vi "UI Loop Main.vi"(10 "UI Panel Ref":T1, 11 "Main Process Class out":refnum<class "Main Class.lvclass">) -> ()   [LabVIEW 2019]
uses:
  Class/Main Process Class/Main Class.lvclass
  LLB/Commonly VI/Ctrl/IDLevel.ctl
  LLB/Commonly VI/Main Glb.vi
  LLB/Message/main/MsgLog.vi
  IO Folder/IO_VI/IOCtrl/Ctrl/IO Card_Type.ctl
  LLB/Message/MsgShowAndLog.lvlib
  LLB/Commonly VI.lvlib
  Axis/Axis_Class/AxisCard.lvclass
  IO Folder/IO_Class/IOCard.lvclass
panel:
  in  "Tab Main 3":refnum<vi>
  in  "Tab Main":refnum<vi>
  out "error out 2":errorcluster
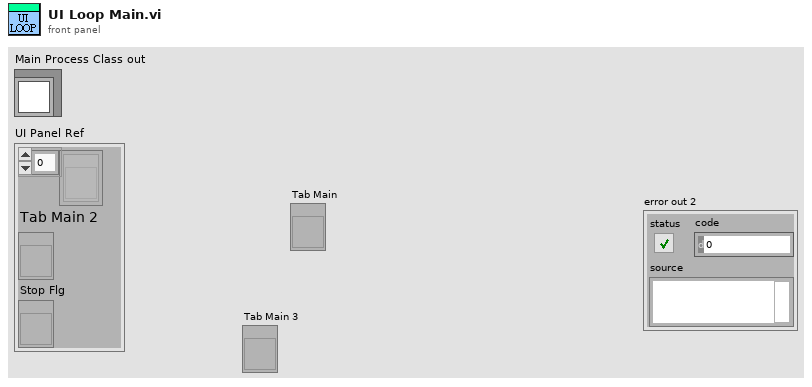
[diagram p1: front panel]
types:
  T1 = cluster{refnum<vi>[], "Tab Main 2":refnum<vi>, "Stop Flg":refnum<vi>}
  T2 = enum16{"initial", "Add", "Write", "Replace", "Delete", "REad"}
  T3 = typedef "IDLevel.ctl" = enum16{"Administrator", "Engineer", "Operator", "LogIn/Out"}
  T4 = typedef "IO Card_Type.ctl" = enum16{"None", "Unidaq32", "6480", "2410C-64", "Zan", "DMC1000B", "16InOut", "Robot", "DMC3600"}
  T5 = enum8{"Enabled", "Disabled", "Disabled and Grayed Out"}
  T6 = typedef "LVPointTypeDef.ctl" = cluster{"Horizontal":i16, "Vertical":i16}
  T7 = cluster{"AutoRunFlg":refnum<vi>, "Action Finish Flg":refnum<vi>, "Remaining Action":refnum<vi>, "Btn_AutoRun":refnum<vi>, "Manual Flg":refnum<vi>, "Sub Process Error":refnum<vi>}
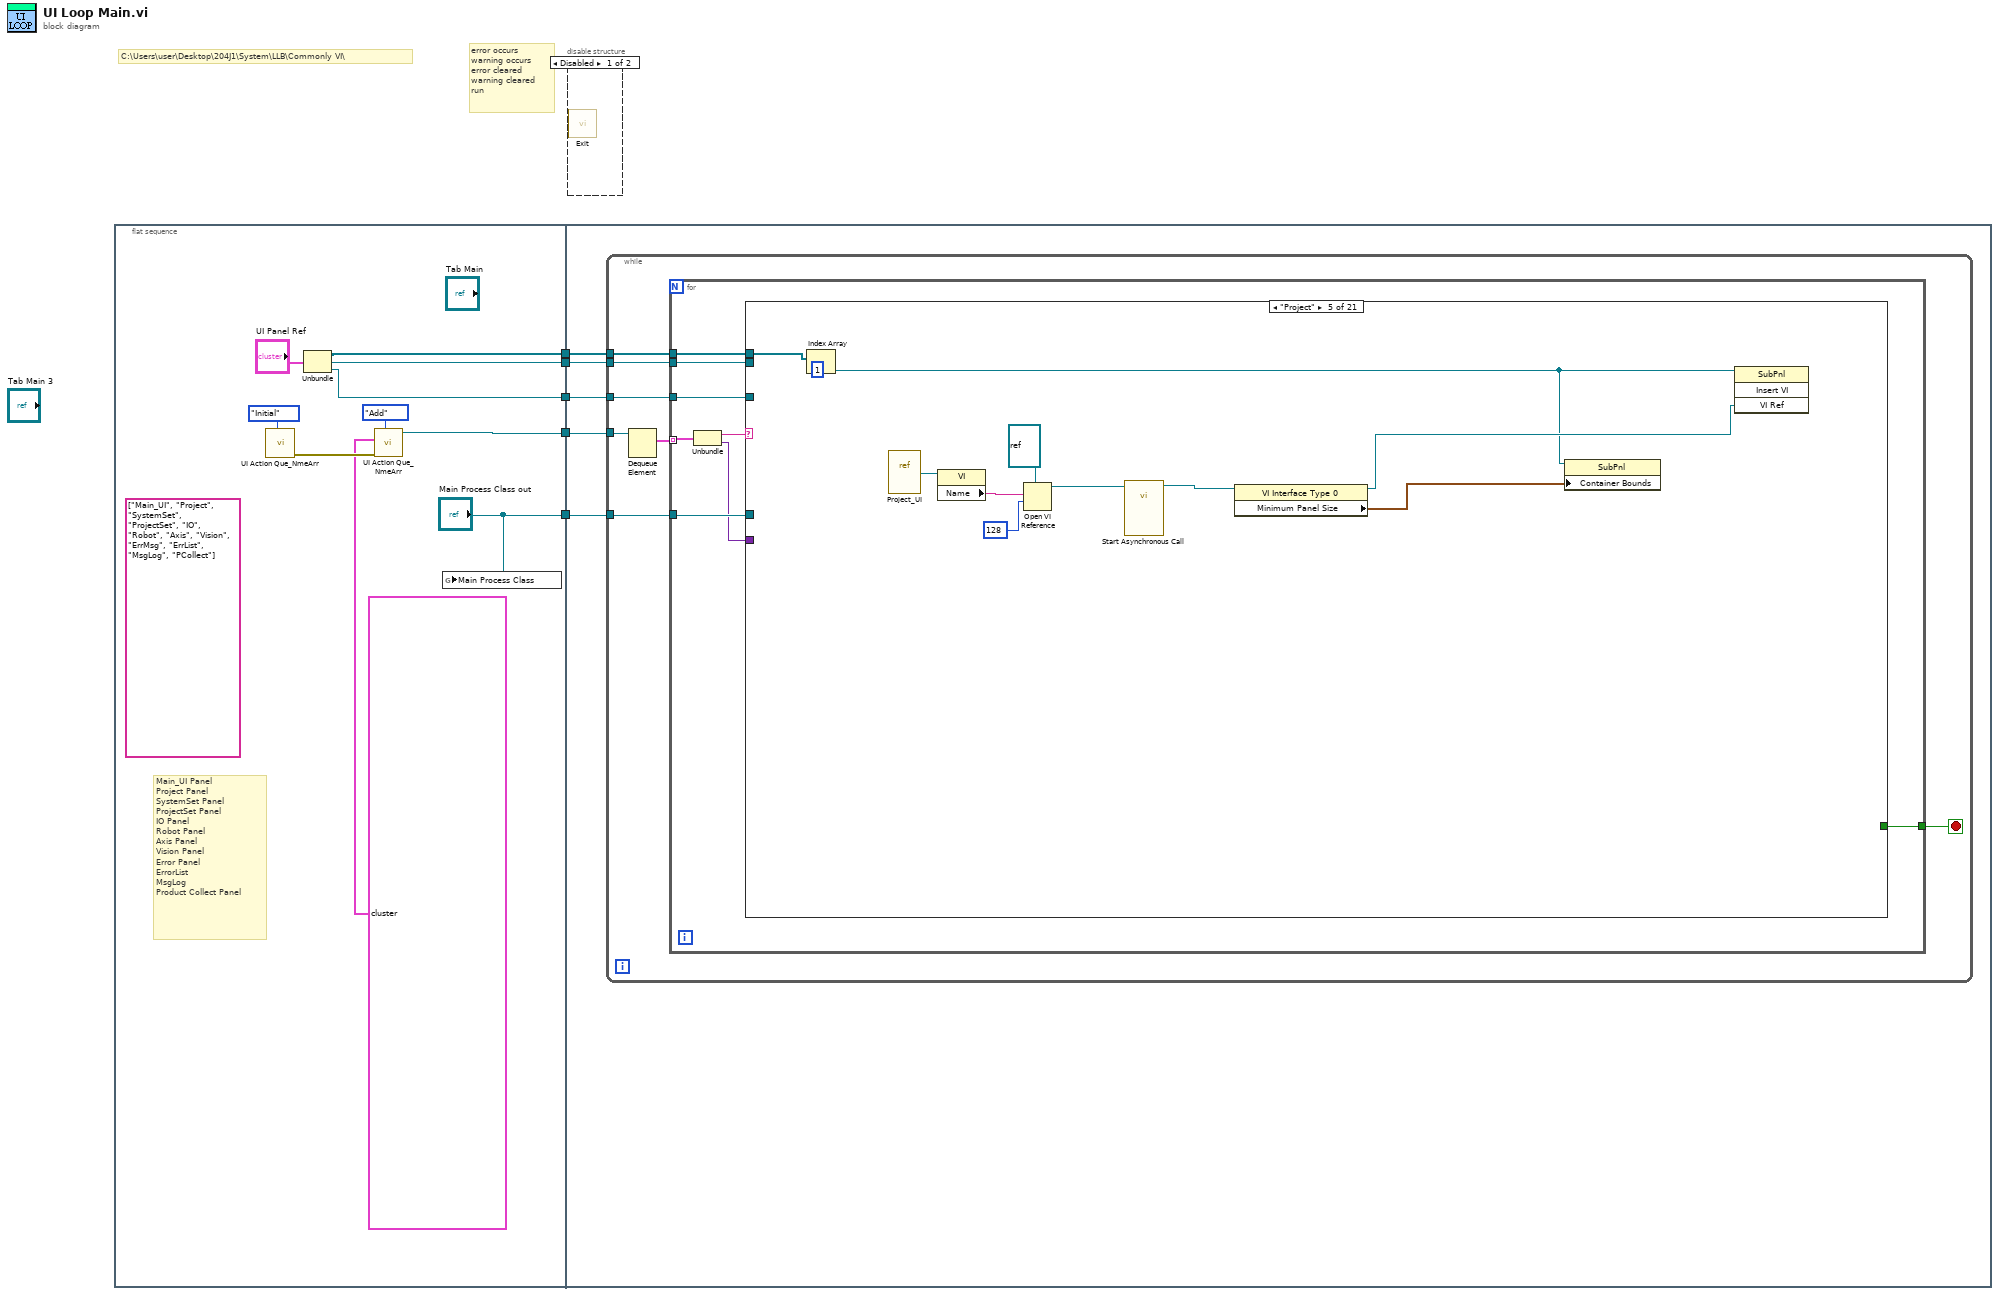
[diagram p0: block diagram]
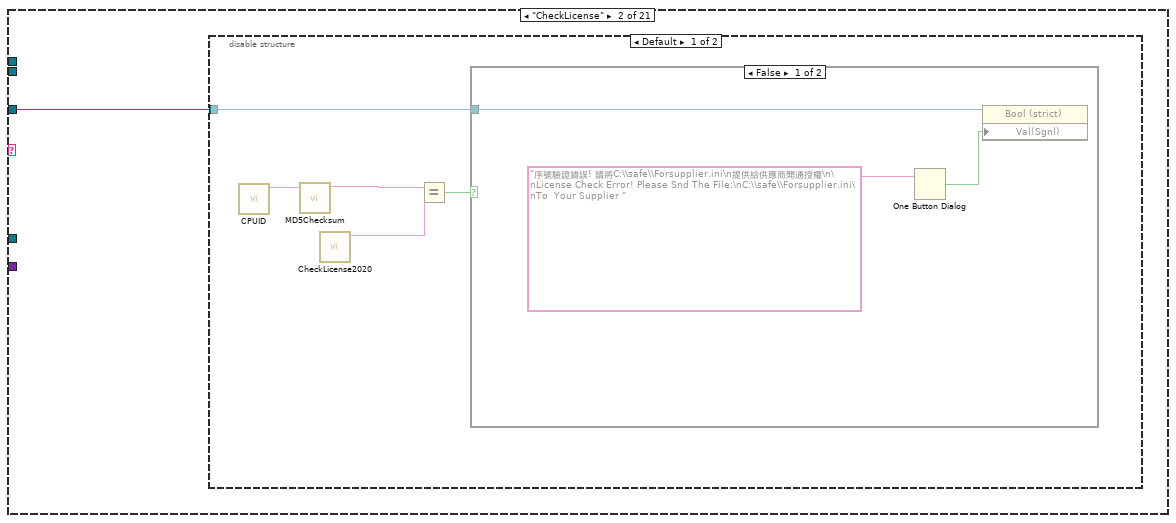
[diagram p4: hidden frame]
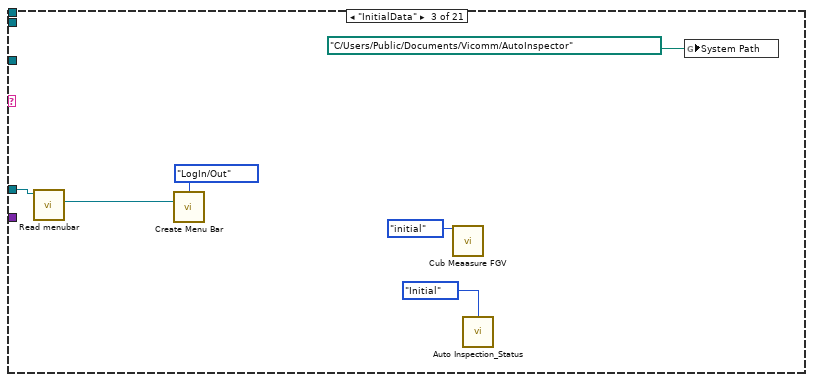
[diagram p7: hidden frame]
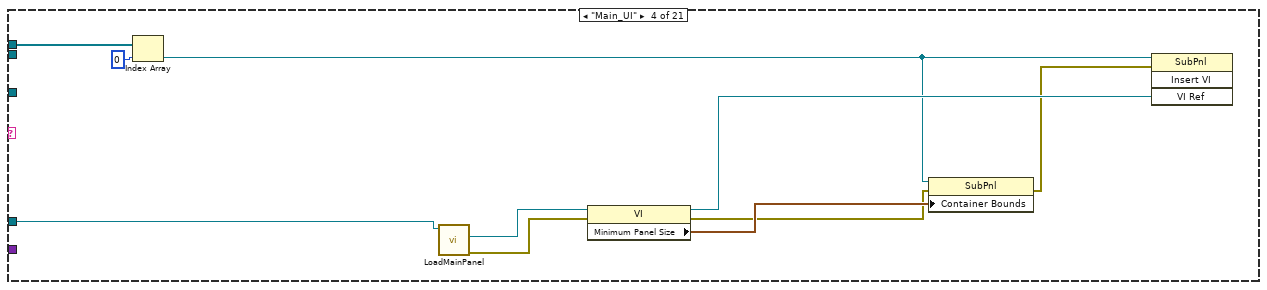
[diagram p8: hidden frame]
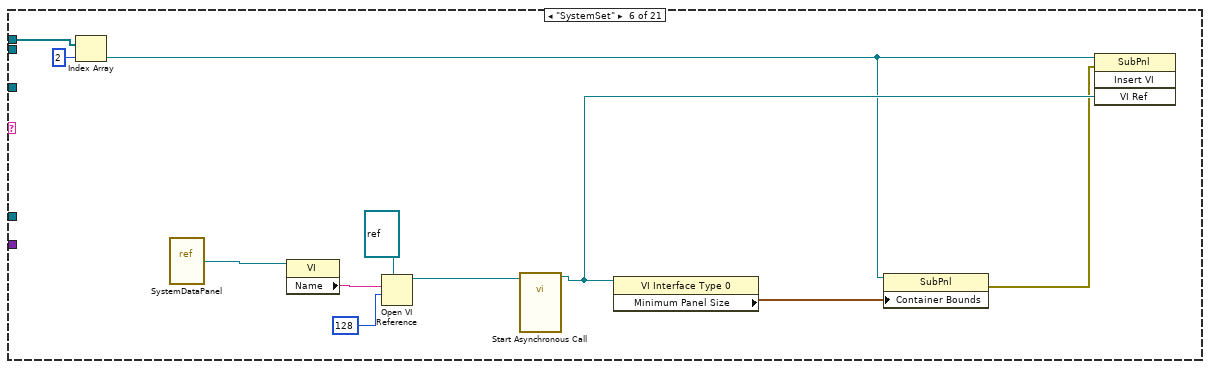
[diagram p9: hidden frame]
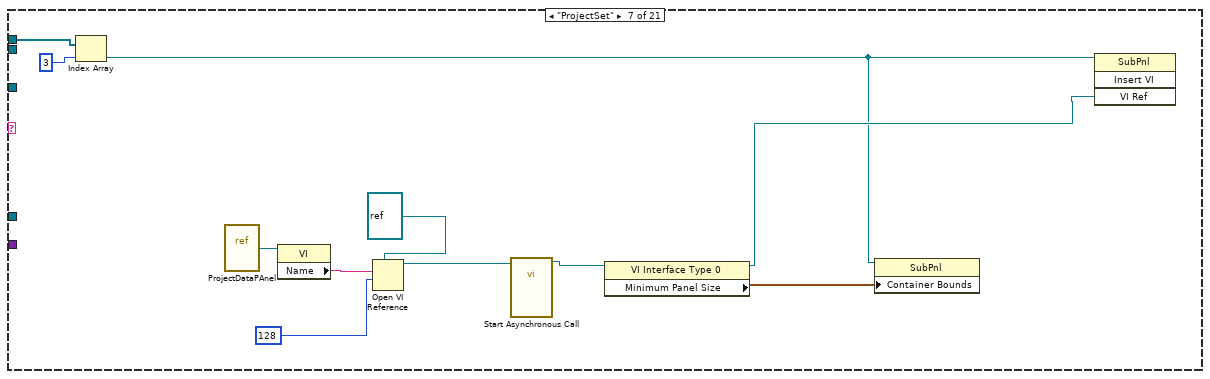
[diagram p10: hidden frame]
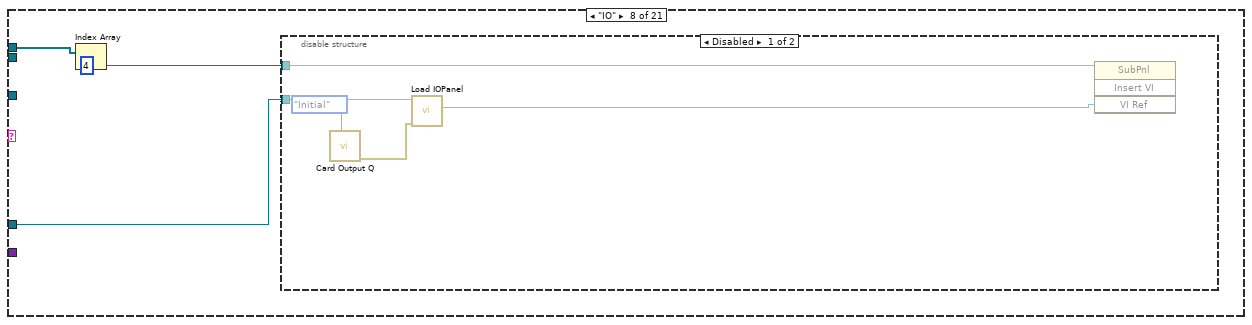
[diagram p11: hidden frame]
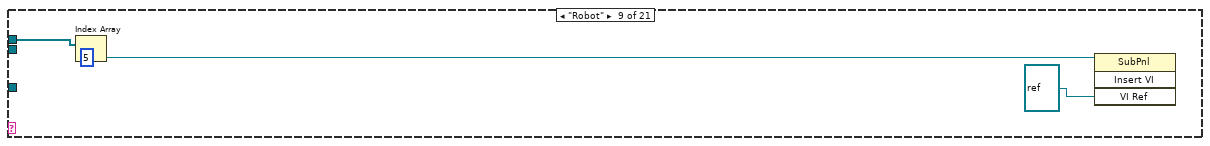
[diagram p13: hidden frame]
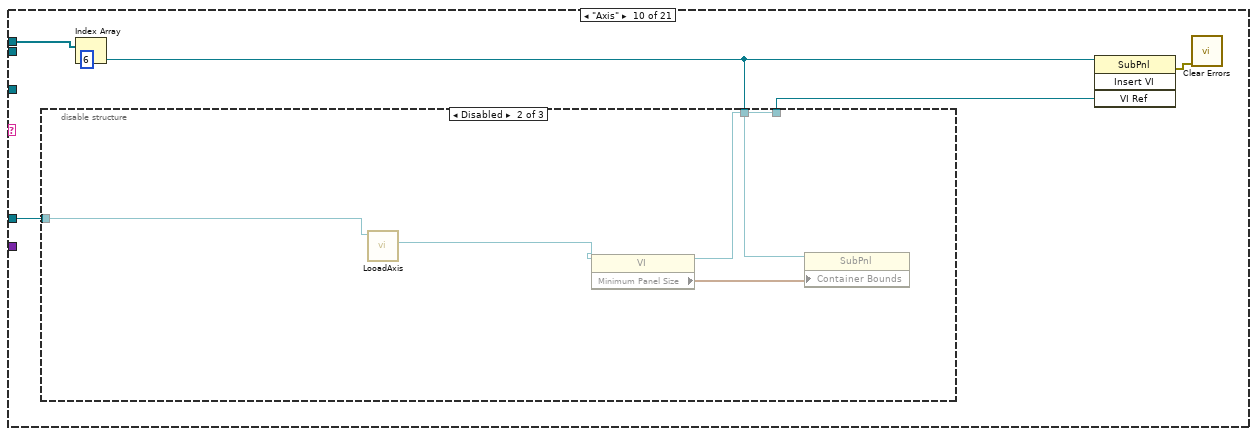
[diagram p14: hidden frame]
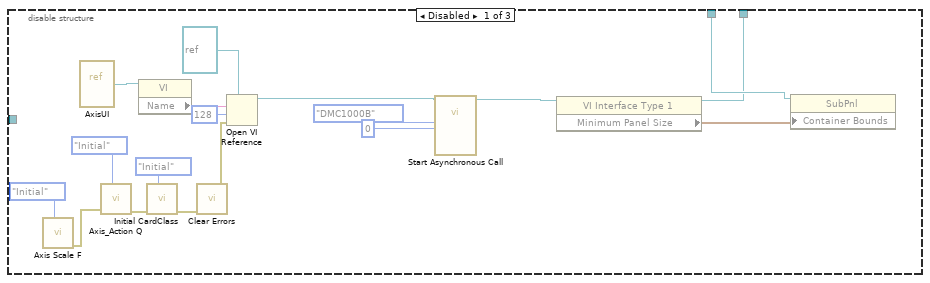
[diagram p15: hidden frame]
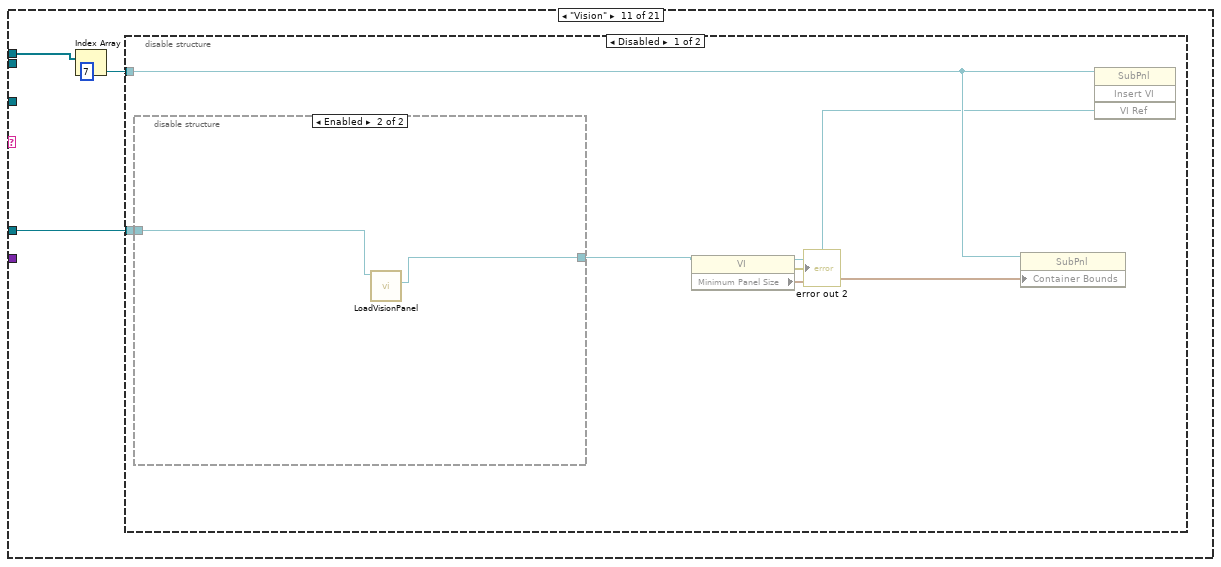
[diagram p17: hidden frame]
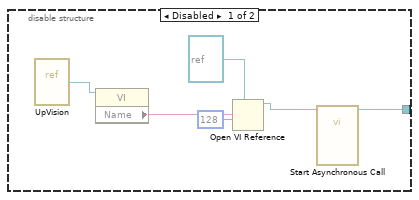
[diagram p18: hidden frame]
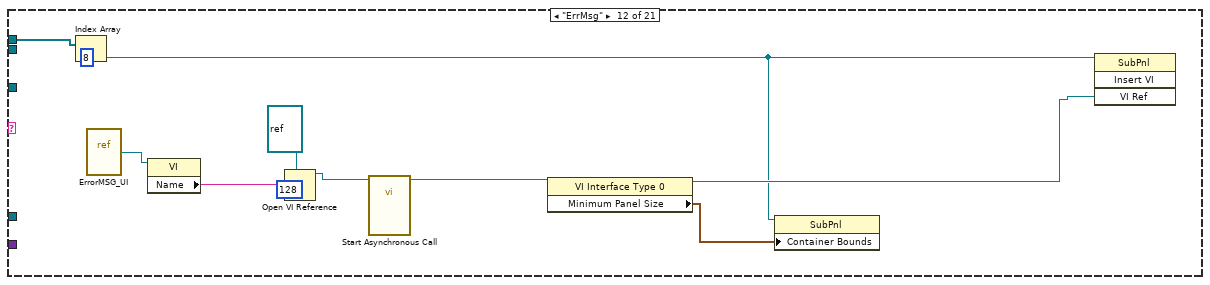
[diagram p20: hidden frame]
diagram:
  # "C:\\Users\\user\\Desktop\\204J1\\System\\LLB\\Commonly VI\\"
  # "error occurs\nwarning occurs\nerror cleared\nwarning cleared\nrun"
  n1 = flat-sequence {
    tunnel: [w13] -> w5
    tunnel: [w9] -> w4
    tunnel: [w8] -> w3
    tunnel: ["Main Process Class out"] -> w2
    tunnel: [w7] -> w1
    tunnel: w5 -> [w20]
    tunnel: w4 -> [w19]
    tunnel: w3 -> [w18]
    tunnel: w2 -> [w17]
    tunnel: w1 -> [w16]
    frame #0 {
      (unwired) string[] ["Main_UI", "Project", "SystemSet", "ProjectSet", "IO", "Robot", "Axis", "Vision", "ErrMsg", "ErrList", "MsgLog", "PCollect"] ("UI Process")
      # "Main_UI Panel\nProject Panel\nSystemSet Panel\nProjectSet Panel\nIO Panel\nRobot Panel\nAxis Panel\nVision Panel\nError Panel\nErrorList\nMsgLog\nProduct Collect Panel"
      n2 = call "UI Action Que_NmeArr.vi"("Action"=enum16{"Initial", "Add", "Release"}."Initial") -> ("error out"=w12:errorcluster)  [unwired: 9 in, 1 out]
      n3 = Unbundle("UI Panel Ref") -> (w9:refnum<vi>[], "Tab Main 2"=w8:refnum<vi>, "Stop Flg"=w7:refnum<vi>)
      n4 = call "UI Action Que_NmeArr.vi"("Action"=enum16{"Initial", "Add", "Release"}."Add", "error in (no error)"=w12, "UI Process"=cluster{"Action":string, "Value":variant}[] [{"Action"="CheckLicense", "Value"=variant}, {"Action"="InitialData", "Value"=variant}, {"Action"="Main_UI", "Value"=variant}, {"Action"="ErrMsg", "Value"=variant}, {"Action"="MsgLog", "Value"=variant}, {"Action"="Project", "Value"=variant}, {"Action"="SystemSet", "Value"=variant}, {"Action"="ProjectSet", "Value"=variant}, {"Action"="IO", "Value"=variant}, {"Action"="Axis", "Value"=variant}, {"Action"="Vision", "Value"=variant}, {"Action"="ErrList", "Value"=variant}, {"Action"="MsgLog", "Value"=variant}, {"Action"="PCollect", "Value"=variant}, {"Action"="Prevention Panel", "Value"=variant}]) -> ("Process Que Out"=w13:refnum<queue>)  [unwired: 7 in, 1 out]
      n5 = global write "Main Glb.vi" "Main Process Class"("Main Process Class out") -> ()
    }
    frame #1 {
      n6 = while {
        tunnel: w20 -> [w27]
        tunnel: w19 -> [w24]
        tunnel: w18 -> [w22]
        tunnel: w17 -> [w23]
        tunnel: w16 -> [w21]
        stop <- w25 stop-if-true
        n7 = Dequeue Element(queue=w27) -> (element=w26:cluster{"Action":string, "Value":variant}[])  [unwired: 2 in, 3 out]
        n8 = for {
          tunnel: w26 -> [w33] mode=indexing
          tunnel: [w35] -> w25
          tunnel: w24 -> [w34]
          tunnel: w23 -> [w31]
          tunnel: w22 -> [w29]
          tunnel: w21 -> [w28]
          n9 = Unbundle(w33) -> ("Action"=w32:string, "Value"=w30:variant)
          n10 = case shown="\"Project\"" w32 {
            tunnel: [_ _ _ _ _ _ _ _ _ _ _ _ _ _ _ _ _ _ _ _ TRUE] -> w35
            tunnel: w34 -> [_ _ _ w60 w70 w81 w92 w95 w104 w111 w138 w163 w171 w183 w195 w204 _ _ _ _ _]
            tunnel: w31 -> [_ _ w49 w55 _ _ _ w94 _ w108 w136 _ w165 _ _ _ w221 _ w230 w236 _]
            tunnel: w30 -> [_ _ _ _ _ _ _ _ _ _ _ _ _ _ _ _ w219 w224 w227 w233 _]
            tunnel: w29 -> [_ _ _ _ _ _ _ _ _ _ _ _ _ _ _ _ w216 w225 _ _ _]
            tunnel: w28 -> [_ w36 _ _ _ _ _ _ _ _ _ _ _ _ _ _ _ _ _ _ _]
            frame Default {
            }
            frame "CheckLicense" {
              n11 = disable-structure shown="Default" {
                disable-tunnel: w36 -> [w41 _]
                frame condition #0 {
                  n12 = call "CPUID.vi"() -> ("ToString"=w40:string)  [unwired: 11 in]
                  n13 = call "MD5Checksum.vi"("Message String"=w40) -> ("MD5 message-digest"=w37:string)  [unwired: 10 in]
                  n14 = call "CheckLicense2020.vi"() -> ("CPU"=w38:string)  [unwired: 11 in]
                  n15 = Equal?(x=w37, y=w38) -> (x = y?=w39:bool)
                  n16 = case shown="False" w39 {
                    tunnel: w41 -> [w44 _]
                    frame False {
                      n17 = One Button Dialog(message="序號驗證錯誤! 請將C:\\safe\\Forsupplier.ini\n提供給供應商開通授權\n\nLicense Check Error! Please Snd The File:\nC:\\safe\\Forsupplier.ini\nTo  Your Supplier ") -> (true=w42:bool)  [unwired: 1 in]
                      n18 = property class="Bool (strict)"(reference=w44, "Val(Sgnl)"=w42) -> ()  [unwired: 1 in, 2 out]
                    }
                    frame True {
                    }
                  }
                }
                frame condition #1 (active) {
                }
              }
            }
            frame "InitialData" {
              n19 = call-dynamic "Read menubar.vi"("Main Class in"=w49) -> ("menubar"=w48:refnum<k9>)  [unwired: 8 in, 2 out]
              n20 = call "Create Menu Bar.vi"("Entry Level"=IDLevel."LogIn/Out", "menubar"=w48) -> ()  [unwired: 13 in, 1 out]
              n21 = call "Cub Meaasure FGV.vi"("Action"=T2."initial" ("Enum")) -> ()  [unwired: 11 in, 8 out]
              n22 = call "Auto Inspection_Status.vi"("Action"=enum16{"Initial", "Write", "Read"}."Initial") -> ()  [unwired: 12 in, 3 out]
              n23 = global write "Main Glb.vi" "System Path"(path "C:/Users/Public/Documents/Vicomm/AutoInspector" ("path")) -> ()
            }
            frame "Main_UI" {
              n24 = Index Array(array=w60, index=0) -> (element=w56:refnum<vi>)
              n25 = call-dynamic "LoadMainPanel.vi"("Main Class in"=w55) -> ("error out"=w54:errorcluster, "This VI"=w51:refnum<vi>)  [unwired: 8 in, 1 out]
              n26 = property class="VI"(reference=w51, error in=w54) -> (reference out=w57:refnum<vi>, error out=w53:errorcluster, "Minimum Panel Size"=w58:T6)
              n27 = property class="SubPnl"(reference=w56, error in=w53, "Container Bounds"=w58) -> (error out=w52:errorcluster)  [unwired: 1 out]
              n28 = invoke class="SubPnl" method="Insert VI"(reference=w56, error in=w52, "VI Ref"=w57) -> ()  [unwired: 1 in, 4 out]
            }
            frame "Project" {
              n29 = Index Array(array=w70, index=1) -> (element=w62:refnum<vi>)
              n30 = vi-ref "Project_UI.vi"() -> (w69:refnum<vi>)
              n31 = property class="VI"(reference=w69) -> ("Name"=w68:string)  [unwired: 1 in, 2 out]
              n32 = Open VI Reference(type specifier VI Refnum (for type only)=refnum<vi> refnum, vi path=w68, options=128) -> (vi reference=w67:refnum<vi>)  [unwired: 3 in, 1 out]
              n33 = call-by-ref "Start Asynchronous Call"(reference=w67) -> (reference out=w66:refnum<vi>)  [unwired: 13 in, 1 out]
              n34 = property class="VI Interface Type 0"(reference=w66) -> (reference out=w63:refnum<vi>, "Minimum Panel Size"=w65:T6)  [unwired: 1 in, 1 out]
              n35 = property class="SubPnl"(reference=w62, "Container Bounds"=w65) -> ()  [unwired: 1 in, 2 out]
              n36 = invoke class="SubPnl" method="Insert VI"(reference=w62, "VI Ref"=w63) -> ()  [unwired: 2 in, 4 out]
            }
            frame "SystemSet" {
              n37 = Index Array(array=w81, index=2) -> (element=w73:refnum<vi>)
              n38 = vi-ref "SystemDataPanel.vi"() -> (w80:refnum<vi>)
              n39 = property class="VI"(reference=w80) -> ("Name"=w79:string)  [unwired: 1 in, 2 out]
              n40 = Open VI Reference(type specifier VI Refnum (for type only)=refnum<vi> refnum, vi path=w79, options=128) -> (vi reference=w78:refnum<vi>)  [unwired: 3 in, 1 out]
              n41 = call-by-ref "Start Asynchronous Call"(reference=w78) -> (reference out=w74:refnum<vi>)  [unwired: 13 in, 1 out]
              n42 = property class="VI Interface Type 0"(reference=w74) -> ("Minimum Panel Size"=w77:T6)  [unwired: 1 in, 2 out]
              n43 = property class="SubPnl"(reference=w73, "Container Bounds"=w77) -> (error out=w72:errorcluster)  [unwired: 1 in, 1 out]
              n44 = invoke class="SubPnl" method="Insert VI"(reference=w73, error in=w72, "VI Ref"=w74) -> ()  [unwired: 1 in, 4 out]
            }
            frame "ProjectSet" {
              n45 = Index Array(array=w92, index=3) -> (element=w84:refnum<vi>)
              n46 = vi-ref "ProjectDataPAnel.vi"() -> (w83:refnum<vi>)
              n47 = property class="VI"(reference=w83) -> ("Name"=w91:string)  [unwired: 1 in, 2 out]
              n48 = Open VI Reference(type specifier VI Refnum (for type only)=refnum<vi> refnum, vi path=w91, options=128) -> (vi reference=w90:refnum<vi>)  [unwired: 3 in, 1 out]
              n49 = call-by-ref "Start Asynchronous Call"(reference=w90) -> (reference out=w88:refnum<vi>)  [unwired: 13 in, 1 out]
              n50 = property class="VI Interface Type 0"(reference=w88) -> (reference out=w85:refnum<vi>, "Minimum Panel Size"=w89:T6)  [unwired: 1 in, 1 out]
              n51 = property class="SubPnl"(reference=w84, "Container Bounds"=w89) -> ()  [unwired: 1 in, 2 out]
              n52 = invoke class="SubPnl" method="Insert VI"(reference=w84, "VI Ref"=w85) -> ()  [unwired: 2 in, 4 out]
            }
            frame "IO" {
              n53 = Index Array(array=w95, index=4) -> (element=w97:refnum<vi>)
              n54 = disable-structure shown="Disabled" {
                disable-tunnel: w97 -> [w102 _]
                disable-tunnel: w94 -> [w101 _]
                frame Disabled {
                  n55 = call "Card Output Q.vi"("Action"=enum16{"Initial", "Write", "Read", "Release"}."Initial") -> ("error Out"=w98:errorcluster)  [unwired: 9 in, 1 out]
                  n56 = call-dynamic "Load IOPanel.vi"("error in (no error)"=w98, "Main Class in"=w101) -> ("This VI"=w100:refnum<vi>)  [unwired: 7 in, 2 out]
                  n57 = invoke class="SubPnl" method="Insert VI"(reference=w102, "VI Ref"=w100) -> ()  [unwired: 2 in, 4 out]
                }
                frame Enabled {
                }
              }
            }
            frame "Robot" {
              n58 = Index Array(array=w104, index=5) -> (element=w106:refnum<vi>)
              n59 = invoke class="SubPnl" method="Insert VI"(reference=w106, "VI Ref"=refnum<vi> refnum) -> ()  [unwired: 2 in, 4 out]
            }
            frame "Axis" {
              n60 = Index Array(array=w111, index=6) -> (element=w110:refnum<vi>)
              n61 = disable-structure shown="Disabled" {
                disable-tunnel: w110 -> [w122 w133 _]
                disable-tunnel: [w120 w132 _] -> w109
                disable-tunnel: w108 -> [_ w135 _]
                frame Disabled {
                  n62 = call "Axis Scale F.vi"("Enum"=enum16{"Initial", "Read"}."Initial") -> ("error Out"=w115:errorcluster)  [unwired: 9 in, 1 out]
                  n63 = vi-ref "AxisUI.vi"() -> (w130:refnum<vi>)
                  n64 = call "Axis_Action Q.vi"("Enum"=enum16{"Initial", "Write", "Read"}."Initial", "error in"=w115) -> ("error out"=w117:errorcluster)  [unwired: 7 in, 2 out]
                  n65 = property class="VI"(reference=w130) -> ("Name"=w129:string)  [unwired: 1 in, 2 out]
                  n66 = call "Initial CardClass.vi"("Enum"=enum16{"Initial", "Write", "Read", "Exit"}."Initial", "error in"=w117) -> ("error Out"=w116:errorcluster)  [unwired: 8 in, 1 out]
                  n67 = call <vilib>:"Clear Errors.vi"("error in (no error)"=w116) -> ("error out"=w113:errorcluster)  [unwired: 5 in, 1 out]
                  n68 = Open VI Reference(type specifier VI Refnum (for type only)=refnum<vi> refnum, vi path=w129, options=128, error in (no error)=w113) -> (vi reference=w126:refnum<vi>)  [unwired: 2 in, 1 out]
                  n69 = call-by-ref "Start Asynchronous Call"(reference=w126, "CardNumber"=0, "IO Card Type"=IO_Card_Type."DMC1000B") -> (reference out=w123:refnum<vi>)  [unwired: 11 in, 1 out]
                  n70 = property class="VI Interface Type 1"(reference=w123) -> (reference out=w120:refnum<vi>, "Minimum Panel Size"=w121:T6)  [unwired: 1 in, 1 out]
                  n71 = property class="SubPnl"(reference=w122, "Container Bounds"=w121) -> ()  [unwired: 1 in, 2 out]
                }
                frame Disabled {
                  n72 = call-dynamic "LooadAxis.vi"("Main Class in"=w135) -> ("This VI"=w131:refnum<vi>)  [unwired: 8 in, 2 out]
                  n73 = property class="VI"(reference=w131) -> (reference out=w132:refnum<vi>, "Minimum Panel Size"=w134:T6)  [unwired: 1 in, 1 out]
                  n74 = property class="SubPnl"(reference=w133, "Container Bounds"=w134) -> ()  [unwired: 1 in, 2 out]
                }
                frame Enabled {
                }
              }
              n75 = invoke class="SubPnl" method="Insert VI"(reference=w110, "VI Ref"=w109) -> (error out=w107:errorcluster)  [unwired: 2 in, 3 out]
              n76 = call <vilib>:"Clear Errors.vi"("error in (no error)"=w107) -> ()  [unwired: 5 in, 2 out]
            }
            frame "Vision" {
              n77 = Index Array(array=w138, index=7) -> (element=w137:refnum<vi>)
              n78 = disable-structure shown="Disabled" {
                disable-tunnel: w137 -> [w143 _]
                disable-tunnel: w136 -> [w141 _]
                frame Disabled {
                  n79 = disable-structure shown="Enabled" {
                    disable-tunnel: [w148 w152] -> w145
                    disable-tunnel: w141 -> [_ w153]
                    frame Disabled {
                      n80 = vi-ref "UpVision.vi"() -> (w151:refnum<vi>)
                      n81 = property class="VI"(reference=w151) -> ("Name"=w150:string)  [unwired: 1 in, 2 out]
                      n82 = Open VI Reference(type specifier VI Refnum (for type only)=refnum<vi> refnum, vi path=w150, options=128) -> (vi reference=w149:refnum<vi>)  [unwired: 3 in, 1 out]
                      n83 = call-by-ref "Start Asynchronous Call"(reference=w149) -> (reference out=w148:refnum<vi>)  [unwired: 13 in, 1 out]
                    }
                    frame Enabled {
                      n84 = call-dynamic "LoadVisionPanel.vi"("Main Class in"=w153) -> ("This VI"=w152:refnum<vi>)  [unwired: 8 in, 2 out]
                    }
                  }
                  n85 = property class="VI"(reference=w145) -> (reference out=w142:refnum<vi>, error out=→"error out 2":errorcluster, "Minimum Panel Size"=w144:T6)  [unwired: 1 in]
                  n86 = property class="SubPnl"(reference=w143, "Container Bounds"=w144) -> ()  [unwired: 1 in, 2 out]
                  n87 = invoke class="SubPnl" method="Insert VI"(reference=w143, "VI Ref"=w142) -> ()  [unwired: 2 in, 4 out]
                }
                frame Enabled {
                }
              }
            }
            frame "ErrMsg" {
              n88 = Index Array(array=w163, index=8) -> (element=w155:refnum<vi>)
              n89 = vi-ref "ErrorMSG_UI.vi"() -> (w162:refnum<vi>)
              n90 = property class="VI"(reference=w162) -> ("Name"=w161:string)  [unwired: 1 in, 2 out]
              n91 = Open VI Reference(type specifier VI Refnum (for type only)=refnum<vi> refnum, vi path=w161, options=128) -> (vi reference=w158:refnum<vi>)  [unwired: 3 in, 1 out]
              n92 = call-by-ref "Start Asynchronous Call"(reference=w158) -> (reference out=w157:refnum<vi>)  [unwired: 13 in, 1 out]
              n93 = property class="VI Interface Type 0"(reference=w157) -> (reference out=w156:refnum<vi>, "Minimum Panel Size"=w154:T6)  [unwired: 1 in, 1 out]
              n94 = property class="SubPnl"(reference=w155, "Container Bounds"=w154) -> ()  [unwired: 1 in, 2 out]
              n95 = invoke class="SubPnl" method="Insert VI"(reference=w155, "VI Ref"=w156) -> ()  [unwired: 2 in, 4 out]
            }
            frame "ErrList" {
              n96 = Index Array(array=w171, index=9) -> (element=w169:refnum<vi>)
              n97 = call-dynamic "LoadAdvancePanel.vi"("Main Class in"=w165) -> ("This VI"=w167:refnum<vi>)  [unwired: 8 in, 2 out]
              n98 = property class="VI"(reference=w167) -> (reference out=w166:refnum<vi>, "Minimum Panel Size"=w170:T6)  [unwired: 1 in, 1 out]
              n99 = property class="SubPnl"(reference=w169, "Container Bounds"=w170) -> (reference out=w168:refnum<vi>)  [unwired: 1 in, 1 out]
              n100 = invoke class="SubPnl" method="Insert VI"(reference=w168, "VI Ref"=w166) -> ()  [unwired: 2 in, 4 out]
            }
            frame "MsgLog" {
              n101 = Index Array(array=w183, index=10) -> (element=w176:refnum<vi>)
              n102 = vi-ref "MsgShowAndLog.lvlib:MsgLog.vi"() -> (w182:refnum<vi>)
              n103 = property class="VI"(reference=w182) -> ("Name"=w181:string)  [unwired: 1 in, 2 out]
              n104 = Open VI Reference(type specifier VI Refnum (for type only)=refnum<vi> refnum, vi path=w181, options=128) -> (vi reference=w179:refnum<vi>)  [unwired: 3 in, 1 out]
              n105 = call-by-ref "Start Asynchronous Call"(reference=w179) -> (reference out=w177:refnum<vi>)  [unwired: 13 in, 1 out]
              n106 = property class="VI Interface Type 2"(reference=w177) -> (reference out=w173:refnum<vi>, "Minimum Panel Size"=w175:T6)  [unwired: 1 in, 1 out]
              n107 = property class="SubPnl"(reference=w176, "Container Bounds"=w175) -> (error out=w174:errorcluster)  [unwired: 1 in, 1 out]
              n108 = invoke class="SubPnl" method="Insert VI"(reference=w176, error in=w174, "VI Ref"=w173) -> ()  [unwired: 1 in, 4 out]
            }
            frame "PCollect" {
              n109 = Index Array(array=w195, index=11) -> (element=w192:refnum<vi>)
              n110 = vi-ref "Table Select 2.vi"() -> (w186:refnum<vi>)
              n111 = disable-structure shown="Disabled" {
                frame Disabled {
                  n112 = vi-ref "Prevention Table.vi"() -> (w197:refnum<vi>)
                  n113 = property class="VI"(reference=w197) -> ("Name"=w203:string)  [unwired: 1 in, 2 out]
                  n114 = Open VI Reference(type specifier VI Refnum (for type only)=refnum<vi> refnum, vi path=w203, options=128) -> (vi reference=w202:refnum<vi>)  [unwired: 3 in, 1 out]
                  n115 = call-by-ref "Start Asynchronous Call"(reference=w202) -> (reference out=w200:refnum<vi>)  [unwired: 13 in, 1 out]
                  n116 = property class="VI Interface Type 0"(reference=w200) -> ("Minimum Panel Size"=w201:T6)  [unwired: 1 in, 2 out]
                  n117 = property class="SubPnl"("Container Bounds"=w201) -> ()  [unwired: 2 in, 2 out]
                }
                frame Enabled {
                }
              }
              n118 = property class="VI"(reference=w186) -> ("Name"=w187:string)  [unwired: 1 in, 2 out]
              n119 = Open VI Reference(type specifier VI Refnum (for type only)=refnum<vi> refnum, vi path=w187, options=128) -> (vi reference=w188:refnum<vi>)  [unwired: 3 in, 1 out]
              n120 = call-by-ref "Start Asynchronous Call"(reference=w188) -> (reference out=w185:refnum<vi>)  [unwired: 13 in, 1 out]
              n121 = property class="VI Interface Type 0"(reference=w185) -> (reference out=w191:refnum<vi>, error out=w193:errorcluster, "Minimum Panel Size"=w194:T6)  [unwired: 1 in]
              n122 = property class="SubPnl"(reference=w192, error in=w193, "Container Bounds"=w194) -> ()  [unwired: 2 out]
              n123 = invoke class="SubPnl" method="Insert VI"(reference=w192, "VI Ref"=w191) -> ()  [unwired: 2 in, 4 out]
            }
            frame "Prevention Panel" {
              n124 = Index Array(array=w204, index=12) -> (element=w213:refnum<vi>)
              n125 = vi-ref "Prevention Table.vi"() -> (w209:refnum<vi>)
              n126 = property class="VI"(reference=w209) -> ("Name"=w210:string)  [unwired: 1 in, 2 out]
              n127 = Open VI Reference(type specifier VI Refnum (for type only)=refnum<vi> refnum, vi path=w210, options=128) -> (vi reference=w211:refnum<vi>)  [unwired: 3 in, 1 out]
              n128 = call-by-ref "Start Asynchronous Call"(reference=w211) -> (reference out=w208:refnum<vi>)  [unwired: 13 in, 1 out]
              n129 = property class="VI Interface Type 0"(reference=w208) -> (reference out=w212:refnum<vi>, error out=w214:errorcluster, "Minimum Panel Size"=w215:T6)  [unwired: 1 in]
              n130 = property class="SubPnl"(reference=w213, error in=w214, "Container Bounds"=w215) -> ()  [unwired: 2 out]
              n131 = invoke class="SubPnl" method="Insert VI"(reference=w213, "VI Ref"=w212) -> ()  [unwired: 2 in, 4 out]
            }
            frame "Error Page Act" {
              n132 = Variant To Data(type="", Variant=w219) -> (data=w218:string)  [unwired: 1 in, 1 out]
              n133 = call-dynamic "Write CurrentAction.vi"("CurrentAction"=w218, "Main Process Class in"=w221) -> ("Main Process Class out"=w217:refnum<class "Main Class.lvclass">)  [unwired: 8 in, 1 out]
              n134 = call-dynamic "UI Page Disply_Error Occur.vi"("Tab Main"=w216, "Main Class in"=w217) -> ()  [unwired: 8 in, 2 out]
            }
            frame "ChangePage" {
              n135 = Variant To Data(type=0, Variant=w224) -> (data=w222:i32)  [unwired: 1 in, 1 out]
              n136 = property class="TabCtl (strict)"(reference=w225, "Value"=w222) -> ()  [unwired: 1 in, 2 out]
            }
            frame "ChangeMenuBar" {
              n137 = call-dynamic "Read menubar.vi"("Main Class in"=w230) -> ("menubar"=w229:refnum<k9>)  [unwired: 8 in, 2 out]
              n138 = Variant To Data(type=IDLevel."Administrator" ("Entry Level"), Variant=w227) -> (data=w226:T3)  [unwired: 1 in, 1 out]
              n139 = call "Create Menu Bar.vi"("Entry Level"=w226, "menubar"=w229) -> ()  [unwired: 13 in, 1 out]
            }
            frame "AutorunEnable" {
              n140 = call-dynamic "Read Main Ref.vi"("Main Process Class in"=w236) -> ("Main Ref"=w235:T7)  [unwired: 8 in, 2 out]
              n141 = Unbundle By Name(w235) -> ("Btn_AutoRun"=w234:refnum<vi>)
              n142 = Variant To Data(type=T5."Enabled" ("Disabled"), Variant=w233) -> (data=w231:T5)  [unwired: 1 in, 1 out]
              n143 = property class="Bool (strict)"(reference=w234, "DisabledEnum"=w231) -> ()  [unwired: 1 in, 2 out]
            }
            frame "Exit" {
            }
          }
        }
      }
    }
  }
  n144 = disable-structure shown="Disabled" {
    frame Disabled {
      n145 = call "Exit.vi"() -> ()  [unwired: 11 in, 1 out]
    }
    frame Enabled {
    }
  }
